vi "Boolean to Color.vi"(1 "Boolean":bool) -> (21 "Color":u32)   [LabVIEW 2016]
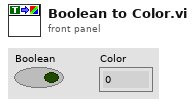
[diagram p1: front panel]
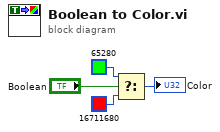
[diagram p0: block diagram]
diagram:
  n1 = Select(t=u32 65280, s="Boolean", f=u32 16711680) -> (s? t:f=→"Color":u32)
